vi "readID.vi"(2 "Buffer Num":u8, 3 "SPI Config In":T1) -> (0 "ID":u32 format="%x", 1 "SPI Config Out":T1)   [LabVIEW 2019]
uses:
  SPI/SPI Config.ctl
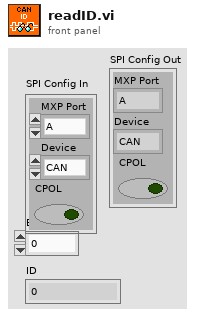
[diagram p1: front panel]
types:
  T1 = typedef "SPI Config.ctl" = cluster{"MXP Port":enum16{"A", "B"}, "Device":enum16{"CAN", "ENC", "IMU1", "IMU2"}, "CPOL":bool}
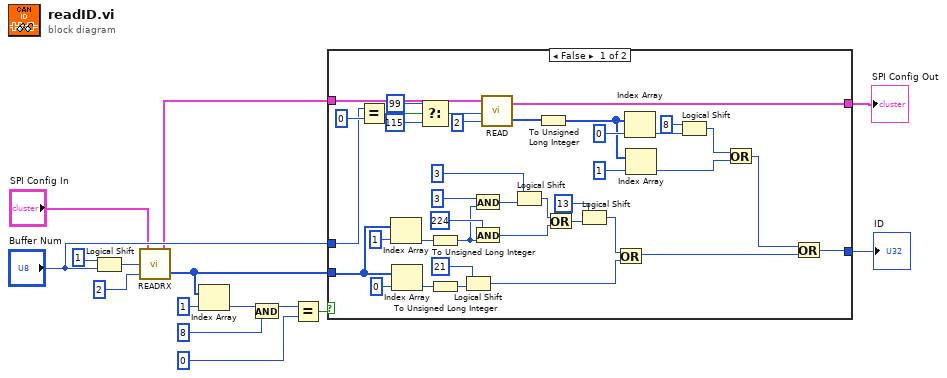
[diagram p0: block diagram]
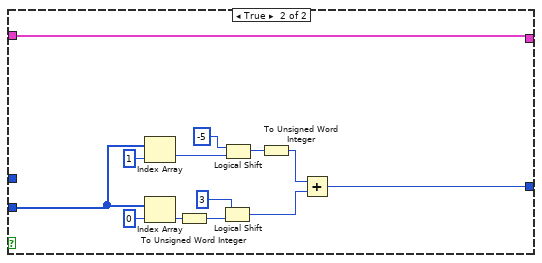
[diagram p2: hidden frame]
diagram:
  n1 = Logical Shift(y=i16 1, x="Buffer Num") -> (x << y=w6:u8)
  n2 = call "READRX.vi"("Registers to Read"=u32 2, "Reg. Select"=w6, "SPI Config In"="SPI Config In") -> ("Data Read"=w4:u8[], "SPI Config Out"=w3:T1)
  n3 = Index Array(array=w4, index=1) -> (element=w13:u8)
  n4 = And(x=w13, y=u8 8) -> (x .and. y?=w11:u8)
  n5 = Equal?(x=w11, y=u8 0) -> (x = y?=w8:bool)
  n6 = case shown="False" w8 {
    tunnel: w4 -> [w51 w56]
    tunnel: [w24 w55] -> w9
    tunnel: "Buffer Num" -> [w35 _]
    tunnel: w3 -> [w17 w54]
    tunnel: [w16 w54] -> w1
    frame False {
      n7 = Equal?(x=w35, y=u8 0) -> (x = y?=w37:bool)
      n8 = Index Array(array=w51, index=1) -> (element=w49:u8)
      n9 = Index Array(array=w51, index=0) -> (element=w50:u8)
      n10 = Select(t=u8 99, s=w37, f=u8 115) -> (s? t:f=w20:u8)
      n11 = To Unsigned Long Integer(number=w49) -> (unsigned 32bit integer=w45:u32)
      n12 = To Unsigned Long Integer(number=w50) -> (unsigned 32bit integer=w48:u32)
      n13 = Logical Shift(y=i16 21, x=w48) -> (x << y=w26:u32)
      n14 = And(x=u32 3, y=w45) -> (x .and. y?=w43:u32)
      n15 = And(x=u32 224, y=w45) -> (x .and. y?=w40:u32)
      n16 = call "READ.vi"("Registers to Read"=u32 2, "Starting Address"=w20, "SPI Config In"=w17) -> ("Frames Read"=w18:u8[], "SPI Config Out"=w16:T1)
      n17 = Logical Shift(y=i16 3, x=w43) -> (x << y=w41:u32)
      n18 = To Unsigned Long Integer(number=w18) -> (unsigned 32bit integer=w21:u32[])
      n19 = Or(x=w41, y=w40) -> (x .or. y?=w34:u32)
      n20 = Logical Shift(y=i16 13, x=w34) -> (x << y=w27:u32)
      n21 = Or(x=w27, y=w26) -> (x .or. y?=w22:u32)
      n22 = Index Array(array=w21, index=0) -> (element=w30:u32)
      n23 = Index Array(array=w21, index=1) -> (element=w25:u32)
      n24 = Logical Shift(y=i16 8, x=w30) -> (x << y=w28:u32)
      n25 = Or(x=w28, y=w25) -> (x .or. y?=w23:u32)
      n26 = Or(x=w23, y=w22) -> (x .or. y?=w24:u32)
    }
    frame True {
      n27 = Index Array(array=w56, index=1) -> (element=w61:u8)
      n28 = Index Array(array=w56, index=0) -> (element=w65:u8)
      n29 = To Unsigned Word Integer(number=w65) -> (unsigned 16bit integer=w64:u16)
      n30 = Logical Shift(y=i16 3, x=w64) -> (x << y=w57:u16)
      n31 = Logical Shift(y=i16 -5, x=w61) -> (x << y=w59:u8)
      n32 = To Unsigned Word Integer(number=w59) -> (unsigned 16bit integer=w58:u16)
      n33 = Add(x=w58, y=w57) -> (x+y=w55:u16)
    }
  }
  "ID" <- w9
  "SPI Config Out" <- w1
